vi "DSF.Engine.Execution.BuilderManager.Get Builders.vi"(8 "error in (no error)":errorcluster, 11 "Builder Manager in":refnum<class "DSF.Engine.Execution.BuilderManager.lvclass">) -> (0 "error out":errorcluster, 2 "Builders":refnum<class "DSF.Engine.Execution.Builder.lvclass">[](array[class]), 3 "Builder Manager out":refnum<class "DSF.Engine.Execution.BuilderManager.lvclass">)   [LabVIEW 2016, in "DSF.Engine.lvlib" / "DSF.Engine.Execution.BuilderManager.lvclass"]
uses:
  DSF.Engine.Execution.BuilderManager.lvclass
  Builder/DSF.Engine.Execution.Builder.lvclass
  DSF.Engine.Execution.BuilderManager.lvclass/DSF.Engine.Execution.BuilderManager.ctl
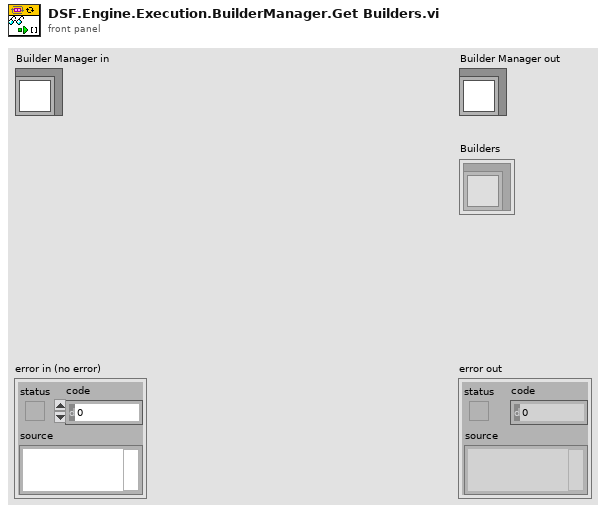
[diagram p1: front panel]
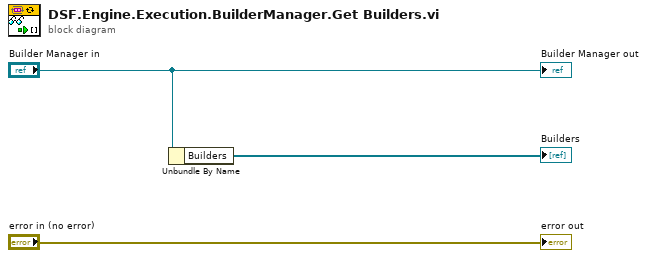
[diagram p0: block diagram]
diagram:
  n1 = Unbundle By Name("Builder Manager in") -> ("Builders"=→"Builders":refnum<class "DSF.Engine.Execution.Builder.lvclass">[])
  "error out" <- "error in (no error)"
  "Builder Manager out" <- "Builder Manager in"
